vi "Instrument.OxfordVRM.SequenceSetMagnetField.vi"(8 "error in (no error)":errorcluster, 10 "Set Magnet Field":T1, 11 "Instrument.Oxford1820":refnum<class "Instrument.OxfordVRM.lvclass">) -> (0 "error out":errorcluster, 3 "Instrument.Oxford1820 out":refnum<class "Instrument.OxfordVRM.lvclass">)   [LabVIEW 2016, in "Instrument.OxfordVRM.lvclass"]
doc: "---------------------------------------------------------------\nJKI State Machine Objects™\nhttp://jki.net/state-machine-objects/\nCopyright (C) 2005-2015, JKI <info@jki.net>\nALL RIGHTS RESERVEDJKI State Machine Objects (SMO) 1.0.0.4\nJKI - JKI\nCopyright (c) 2015, JKI"
uses:
  Instrument.OxfordVRM.lvclass
  Typedefs/PrivateEvents--Instrument.OxfordVRM.SequenceSetMagnetField.ctl
  Typedefs/Instrument.VRM.setMagnet-cluster.ctl
  Typedefs/VRM Targets--Cluster.ctl
  Typedefs/VRM Magnet Axis--Enum.ctl
  Instrument.OxfordVRM.lvclass/Instrument.OxfordVRM.ctl
panel:
  # "For instructions on how to use the JKI State Machine Objects, examples and video tutorials, visit:\nhttp://jki.net/state-machine-objects/\n\nJKI State Machine Objects™\nhttp://jki.net/state-machine-objects/\nCopyright (C) 2005-2015, JKI <info@jki.net>\nALL RIGHTS RESERVED"
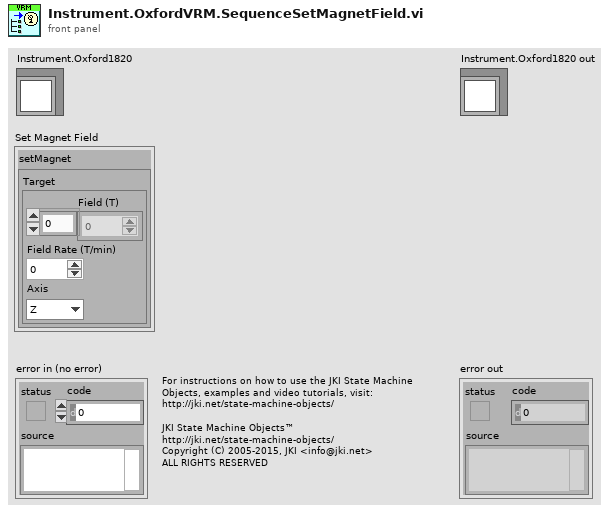
[diagram p1: front panel]
types:
  T1 = typedef "Instrument.OxfordVRM.lvclass/PrivateEvents--Instrument.OxfordVRM.SequenceSetMagnetField.ctl" = cluster{"setMagnet":T2}
  T2 = typedef "Instrument.OxfordVRM.lvclass/Instrument.VRM.setMagnet-cluster.ctl" = cluster{"Target":T3}
  T3 = typedef "Instrument.OxfordVRM.lvclass/VRM Targets--Cluster.ctl" = cluster{"Field (T)":dbl[], "Field Rate (T/min)":dbl, "Axis":T4}
  T4 = typedef "Instrument.OxfordVRM.lvclass/VRM Magnet Axis--Enum.ctl" = enum16{"Z", "X", "Y", "ALL"}
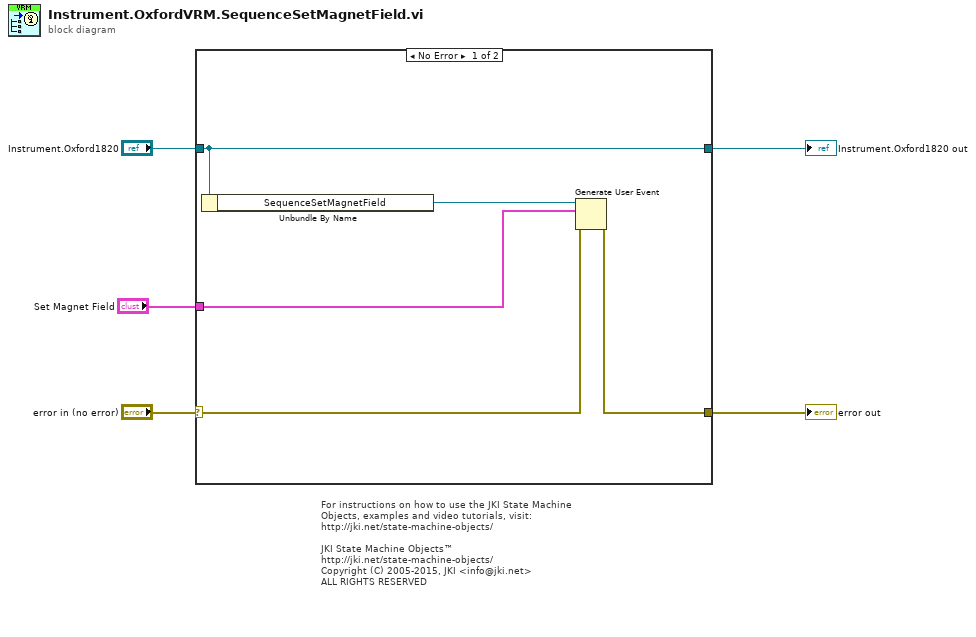
[diagram p0: block diagram]
diagram:
  # "For instructions on how to use the JKI State Machine Objects, examples and video tutorials, visit:\nhttp://jki.net/state-machine-objects/\n\nJKI State Machine Objects™\nhttp://jki.net/state-machine-objects/\nCopyright (C) 2005-2015, JKI <info@jki.net>\nALL RIGHTS RESERVED"
  n1 = case shown="No Error" "error in (no error)" {
    selector: "error in (no error)" -> [w10 w12]
    tunnel: [w8 w12] -> w4
    tunnel: [w7 w11] -> w5
    tunnel: "Instrument.Oxford1820" -> [w7 w11]
    tunnel: "Set Magnet Field" -> [w6 _]
    frame No Error {
      n2 = Unbundle By Name(w7) -> ("SequenceSetMagnetField"=w9:refnum<user-event>)
      n3 = Generate User Event(user event=w9, event data cluster=w6, error in=w10) -> (error out=w8:errorcluster)  [unwired: 1 in, 1 out]
    }
    frame Error {
    }
  }
  "error out" <- w4
  "Instrument.Oxford1820 out" <- w5
